vi "Verify Dispatcher Queue.vi"(0 "receiver host (\"\")":string, 5 "receiver port (0)":u16, 7 "queue name":string, 9 "timeout (100 ms)":i32=100, 11 "error in":errorcluster) -> (4 "response message":T1, 6 "string response":string, 15 "error out":errorcluster)   [LabVIEW 2009, in "AMC.lvlib"]
doc: "Requests confirmation that the spefcified queue name exists in the application instance specified by \"receiver host\" and \"receiver port\".\n\nIf \"receiver port\" is undefined, this VI will attempt to use the default UDP port."
uses:
  AMC.lvlib
  Message.ctl
  <vilib>/NI/Tools/Keyed Array/KeyedArray.ctl
  Globals.vi
  <vilib>/NI/Tools/Keyed Array/Tools_KeyedArray.lvlib
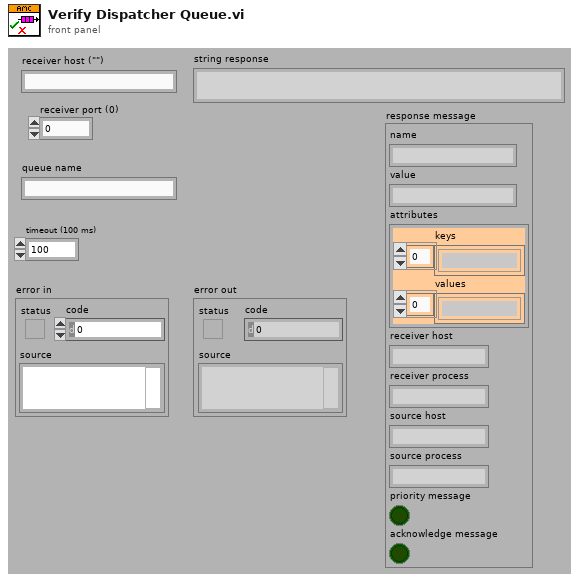
[diagram p1: front panel]
types:
  T1 = typedef "AMC.lvlib/Message.ctl" = cluster{"name":string, "value":string, "attributes":T2, "receiver host":string, "receiver process":string, "source host":string, "source process":string, "priority message":bool, "acknowledge message":bool}
  T2 = typedef "Tools_KeyedArray.lvlib/KeyedArray.ctl" = cluster{"keys":string[], "values":string[]}
  T3 = typedef "AMC.lvlib/Message Queue.ctl" = refnum<queue>
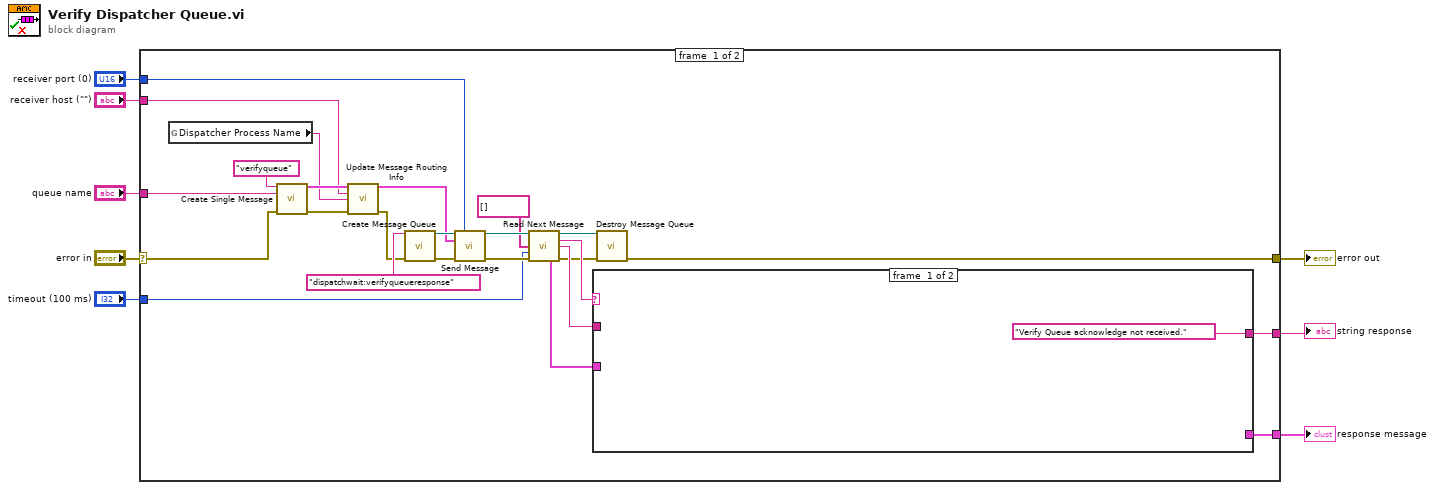
[diagram p0: block diagram]
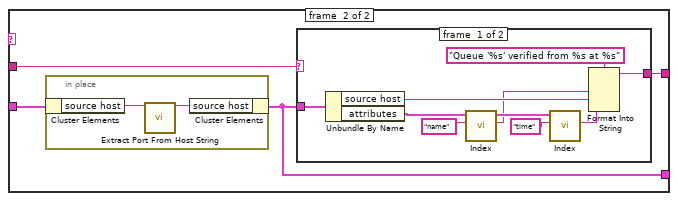
[diagram p2: hidden frame]
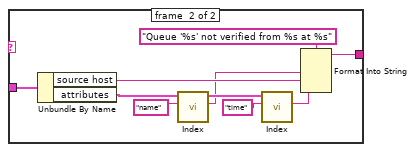
[diagram p3: hidden frame]
diagram:
  n1 = case shown="No Error" "error in" {
    selector: "error in" -> [w15 w61]
    tunnel: [w33 _] -> w8
    tunnel: [w32 _] -> w7
    tunnel: [w31 w61] -> w6
    tunnel: "queue name" -> [w24 _]
    tunnel: "receiver host (\"\")" -> [w18 _]
    tunnel: "timeout (100 ms)" -> [w10 _]
    tunnel: "receiver port (0)" -> [w11 _]
    frame #0 {
      n2 = global read "Globals.vi" "Dispatcher Process Name"() -> (w17:string)
      n3 = call "Create Single Message.vi"("name"="verifyqueue" ("Name"), "value"=w24, "error in"=w15) -> ("message"=w20:T1, "error out"=w16:errorcluster)  [unwired: 11 in]
      n4 = call "Update Message Routing Info.vi"("message"=w20, "receiver host (\"\")"=w18, "receiver process (\"\")"=w17, "error in"=w16) -> ("message"=w19:T1, "error out"=w14:errorcluster)  [unwired: 10 in]
      n5 = call "Create Message Queue.vi"("message queue name"="dispatchwait:verifyqueueresponse", "error in"=w14) -> ("message queue out"=w27:T3, "error out"=w29:errorcluster)  [unwired: 12 in]
      n6 = call "Send Message.vi"("message queue in"=w27, "receiver port (0)"=w11, "message"=w19, "error in"=w29) -> ("message queue out"=w26:T3, "error out"=w30:errorcluster)  [unwired: 9 in, 1 out]
      n7 = call "Read Next Message.vi"("message queue in"=w26, "termination list ([Exit])"=string[] [], "timeout (1 ms)"=w10, "error in"=w30) -> ("message queue out"=w12:T3, "message name"=w23:string, "message value"=w22:string, "message"=w21:T1, "error out"=w13:errorcluster)  [unwired: 4 in, 3 out]
      n8 = case shown="\"verifyqueueack\"" w23 {
        tunnel: w21 -> [_ w36]
        tunnel: ["Verify Queue acknowledge not received." w38] -> w33
        tunnel: [_ w35] -> w32
        tunnel: w22 -> [_ w37]
        frame #0 {
        }
        frame #1 {
          n9 = in-place {
            n10 = in-place-cluster #1(w36) -> ("source host"=w40:string)
            n11 = call "Extract Port From Host String.vi"("host in"=w40) -> ("host out"=w39:string)  [unwired: 12 in, 2 out]
            n12 = in-place-cluster #1("source host"=w39) -> (w35:T1)
          }
          n13 = case shown="\"ok\"" w37 {
            tunnel: [w46 w56] -> w38
            tunnel: w35 -> [w45 w55]
            frame #0 {
              n14 = Unbundle By Name(w45) -> ("source host"=w50:string, "attributes"=w43:T2)
              n15 = call <vilib>:"Index.vi"("key"="name", "array in"=w43) -> ("value"=w41:string, "duplicate array"=w42:T2)  [unwired: 2 in, 2 out]
              n16 = call <vilib>:"Index.vi"("key"="time", "array in"=w42) -> ("value"=w49:string)  [unwired: 2 in, 3 out]
              n17 = Format Into String(format string="Queue '%s' verified from %s at %s", w41, w50, w49) -> (resulting string=w46:string)  [unwired: 2 in, 1 out]
            }
            frame #1 {
              n18 = Unbundle By Name(w55) -> ("source host"=w60:string, "attributes"=w53:T2)
              n19 = call <vilib>:"Index.vi"("key"="name", "array in"=w53) -> ("value"=w51:string, "duplicate array"=w52:T2)  [unwired: 2 in, 2 out]
              n20 = call <vilib>:"Index.vi"("key"="time", "array in"=w52) -> ("value"=w59:string)  [unwired: 2 in, 3 out]
              n21 = Format Into String(format string="Queue '%s' not verified from %s at %s", w51, w60, w59) -> (resulting string=w56:string)  [unwired: 2 in, 1 out]
            }
          }
        }
      }
      n22 = call "Destroy Message Queue.vi"("message queue in"=w12, "error in"=w13) -> ("error out"=w31:errorcluster)  [unwired: 11 in, 2 out]
    }
    frame #1 {
    }
  }
  "error out" <- w6
  "string response" <- w8
  "response message" <- w7
